vi "Main.vi"() -> ()   [LabVIEW 2016]
uses:
  <vilib>/Utility/file.llb/Read Delimited Spreadsheet (string).vi
panel:
  in  "Reset":bool
  in  "Base Path for Relative Source Path":path
  out "Progress":i32(slide) scale=0.0..4.0
  out "Error Out":errorcluster
  out "Done?":bool
  in  "Copy Folders":bool
  in  "Configuration File Path (Tab Delimited File)":path
  # "Copy Folders v0.1"
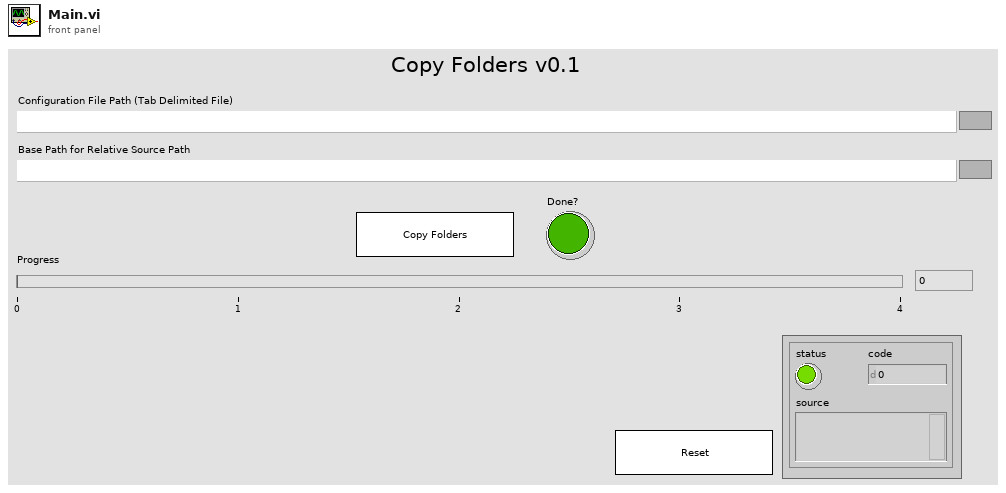
[diagram p1: front panel]
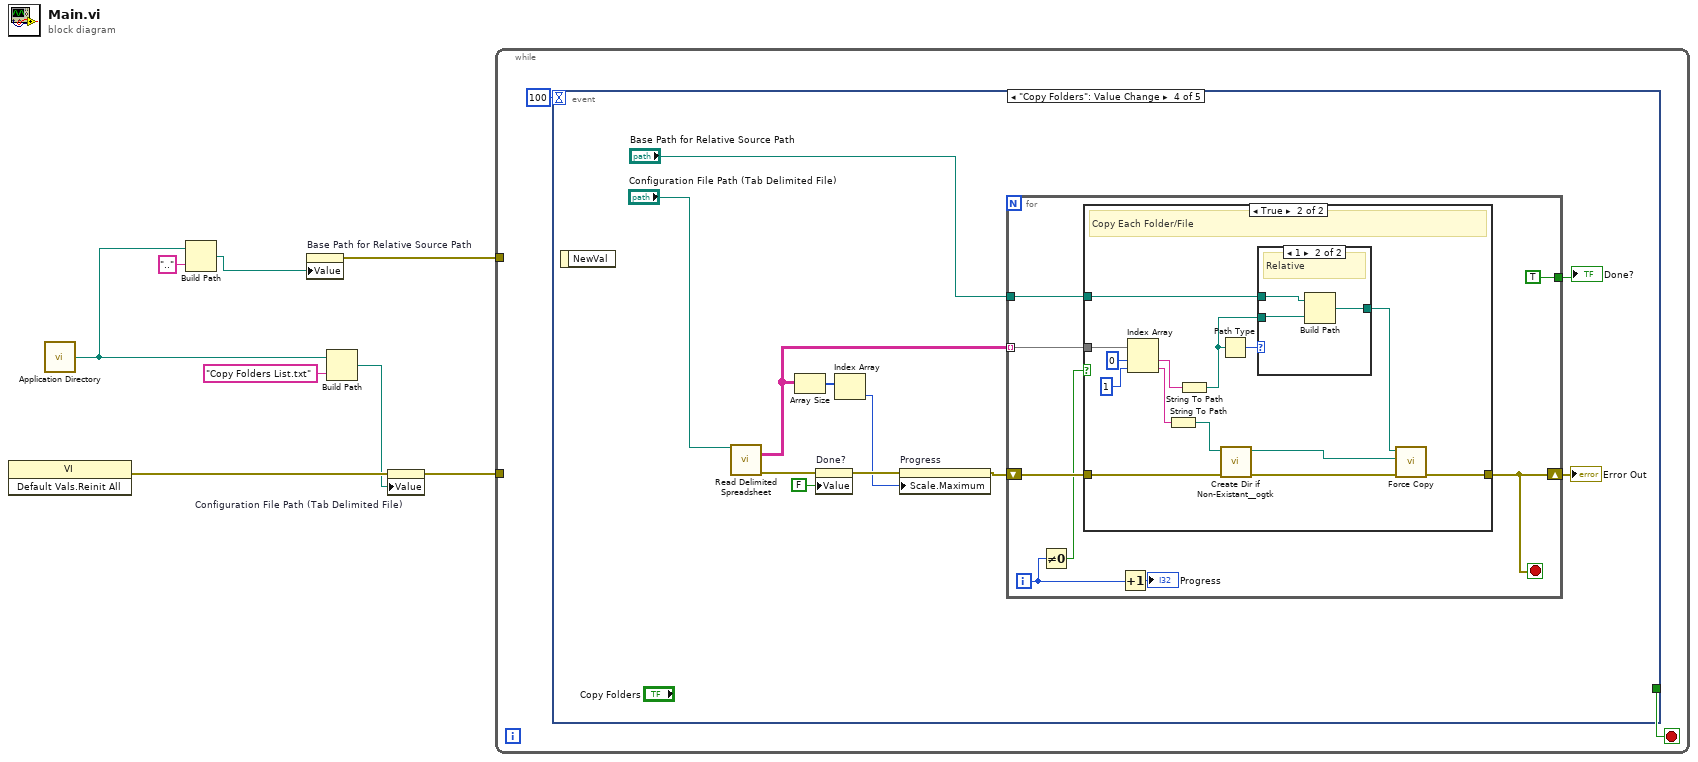
[diagram p0: block diagram]
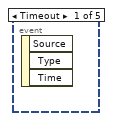
[diagram p2: hidden frame]
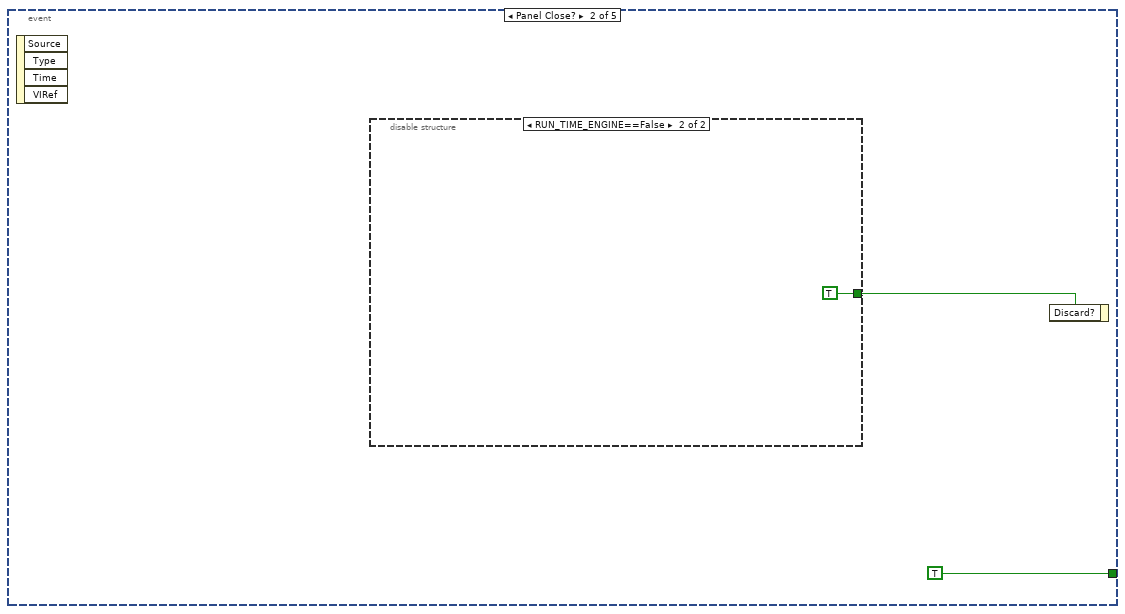
[diagram p3: hidden frame]
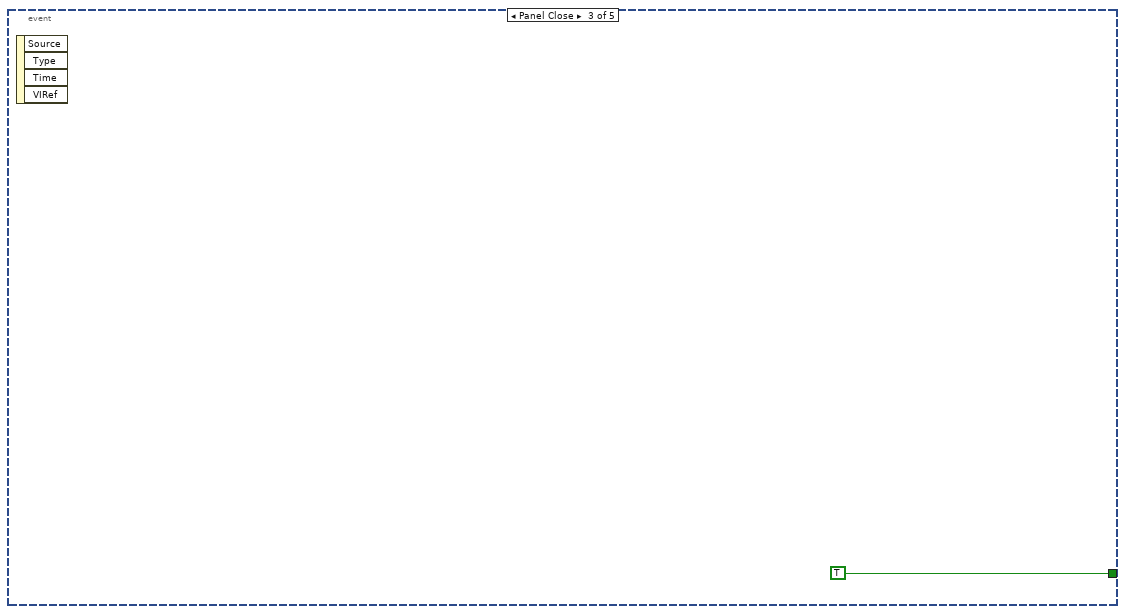
[diagram p5: hidden frame]
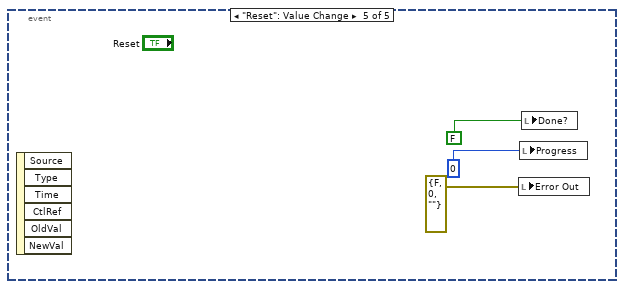
[diagram p8: hidden frame]
diagram:
  n1 = invoke class="VI" method="Default Vals.Reinit All"() -> (error out=w8:errorcluster)  [unwired: 3 in, 2 out]
  n2 = call <vilib>:"Application Directory.vi"() -> ("Application Directory"=w3:path)
  n3 = Build Path(base path=w3, name or relative path="..") -> (appended path=w1:path)
  n4 = property on="Base Path for Relative Source Path" class="Path"("Value"=w1) -> (error out=w4:errorcluster)  [unwired: 2 in, 1 out]
  n5 = Build Path(base path=w3, name or relative path="Copy Folders List.txt") -> (appended path=w5:path)
  n6 = property on="Configuration File Path (Tab Delimited File)" class="Path"(error in=w8, "Value"=w5) -> (error out=w7:errorcluster)  [unwired: 1 in, 1 out]
  n7 = while {
    tunnel: w7 -> [_]
    tunnel: w4 -> [_]
    stop <- w9 stop-if-true
    n8 = event shown="[3] \"Copy Folders\": Value Change" {
      selector: _ -> [_ _ _ _ _]
      dyn-events: _ -> [_ _ _ _ _]
      timeout: 100 -> [_ _ _ _ _]
      tunnel: [_ TRUE TRUE _ _] -> w9
      event Timeout {
        n9 = event-data() -> ()  [unwired: 1 in, 3 out]
      }
      event Panel Close? {
        n10 = event-data() -> ()  [unwired: 1 in, 4 out]
        n11 = disable-structure shown="RUN_TIME_ENGINE==False" {
          disable-tunnel: [_ TRUE] -> w12
          frame condition #0 {
          }
          frame condition #1 (active) {
          }
        }
        n12 = event-data("Discard?"=w12) -> ()  [unwired: 1 in, 1 out]
      }
      event Panel Close {
        n13 = event-data() -> ()  [unwired: 1 in, 4 out]
      }
      event "Copy Folders": Value Change {
        n14 = event-data() -> ()  [unwired: 1 in, 1 out]
        n15 = call-poly <vilib>:"Read Delimited Spreadsheet.vi"("file path (dialog if empty)"="Configuration File Path (Tab Delimited File)") -> ("all rows"=w18:string[][], "error out"=w23:errorcluster)  [unwired: 9 in, 4 out]
        n16 = Array Size(array=w18) -> (size(s)=w17:i32[])
        n17 = property on="Done?" class="Bool (strict)"(error in=w23, "Value"=FALSE ("Done?")) -> (error out=w20:errorcluster)  [unwired: 1 in, 1 out]
        n18 = Index Array(array=w17) -> (element=w16:i32)  [unwired: 1 in]
        n19 = property on="Progress" class="Slide (strict)"(error in=w20, "Scale.Maximum"=w16) -> (error out=w19:errorcluster)  [unwired: 1 in, 1 out]
        n20 = for {
          tunnel: w18 -> [w33] mode=indexing
          tunnel: [TRUE] -> w24
          shift-right: [w31] -> w22
          shift-left: w19 -> [w29]
          tunnel: "Base Path for Relative Source Path" -> [w28]
          i -> [w27]
          stop <- w31 stop-if-true
          n21 = Not Equal To 0?(x=w27) -> (x != 0?=w26:bool)
          n22 = case shown="True" w26 {
            tunnel: w33 -> [_ w48]
            tunnel: [w34 w43] -> w31
            tunnel: w29 -> [w34 w42]
            tunnel: w28 -> [_ w37]
            frame False {
              # "Ignore Headers"
            }
            frame True {
              # "Copy Each Folder/File"
              n23 = Index Array(array=w48, index #1=0 ("index"), index #2=1 ("index")) -> (element #1=w45:string, element #2=w44:string)
              n24 = String To Path(string=w44) -> (path=w40:path)
              n25 = String To Path(string=w45) -> (path=w36:path)
              n26 = Path Type(1:w36) -> (0:w38:i16)
              n27 = call <userlib>:"Create Dir if Non-Existant__ogtk.vi"("error in (no error)"=w42, "Directory Path"=w40) -> ("error out"=w41:errorcluster, "dup Directory Path"=w39:path)  [unwired: 7 in, 1 out]
              n28 = case shown="1" w38 {
                tunnel: w37 -> [_ w52]
                tunnel: w36 -> [w49 w51]
                tunnel: [w49 w50] -> w35
                frame 0, Default {
                }
                frame 1 {
                  # "Relative"
                  n29 = Build Path(base path=w52, name or relative path=w51) -> (appended path=w50:path)
                }
              }
              n30 = call "Force Copy.vi"("error in (no error)"=w41, "target"=w39, "source"=w35) -> ("error out"=w43:errorcluster)  [unwired: 8 in]
            }
          }
          n31 = Increment(x=w27) -> (x+1=→"Progress":i32)
        }
        "Done?" <- w24
        "Error Out" <- w22
      }
      event "Reset": Value Change {
        n32 = event-data() -> ()  [unwired: 1 in, 6 out]
        n33 = local write "Error Out"(errorcluster {"status"=FALSE, "code"=0, "source"=""} ("Error Out")) -> ()
        n34 = local write "Progress"(0 ("Progress")) -> ()
        n35 = local write "Done?"(FALSE ("Done?")) -> ()
      }
    }
  }
